vi "AddTopProcessRun.vi"(5 "ProcessRunStartTime (Now)":timestamp, 6 "ProcessRunStatus (NOT_COMPLETED)":T1=enum."NOT_COMPLETED", 7 "ProductFullName (Generic_Product)":string="Generic_Product", 8 "error in":errorcluster, 9 "ProductUnitIdentifier":string, 10 "ProcessFullName (Generic_Process)":string="Generic_Process", 11 "Datawarehouse in":refnum<class "Datawarehouse.lvclass">) -> (0 "error out":errorcluster, 2 "TopProcessRun":refnum<class "ProcessRun.lvclass">, 3 "Datawarehouse out":refnum<class "Datawarehouse.lvclass">)   [LabVIEW 2021, in "ProligentXMLGenerator.lvlib" / "Datawarehouse.lvclass"]
doc: "Add a Top Process Run.\n\nDefines a process run, a logical container for the execution of operations. Process runs are globaly unique by their ProcessRunId property."
uses:
  Datawarehouse.lvclass
  Datawarehouse.lvclass/Datawarehouse.ctl
  ProcessRun/ProcessRun.lvclass
  Base/ExecutionStatus/Value.ctl
  Base/ExecutionStatus/ExecutionStatus.lvclass
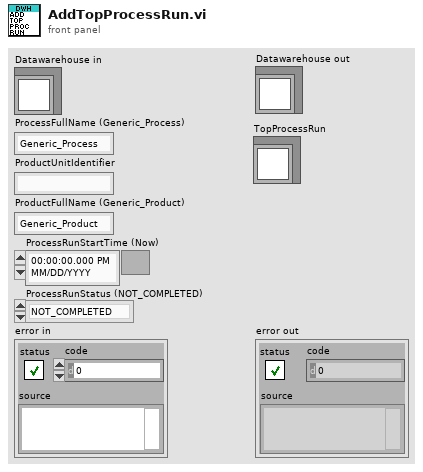
[diagram p1: front panel]
types:
  T1 = typedef "ProligentXMLGenerator.lvlib/ExecutionStatus.lvclass/Value.ctl" = enum16{"PASS", "FAIL", "NOT_COMPLETED", "ABORTED"}
  T2 = typedef "ProligentXMLGenerator.lvlib/Datawarehouse.lvclass/Data.ctl" = cluster{"DestinationFolder":path, "BaseFileName":string, "Document":refnum<k20>, "Defects":refnum<class "Defect.lvclass">[], "TopProcessRuns":refnum<class "ProcessRun.lvclass">[], "ProductUnits":refnum<class "ProductUnit.lvclass">[], "GenerationTime":refnum<class "DateTime.lvclass">, "DataSourceFingerprint":refnum<class "NonEmptyString_448.lvclass">, "IntegrationMetaData":refnum<class "NonEmptyString_2000.lvclass">, "TimeZoneInfoId":string}
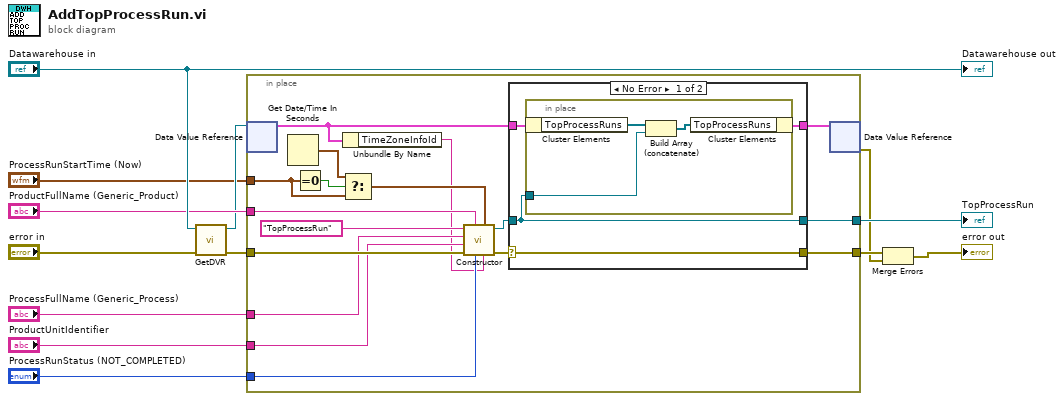
[diagram p0: block diagram]
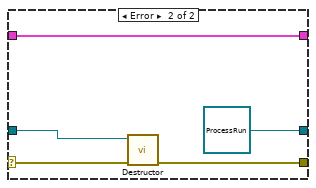
[diagram p2: hidden frame]
diagram:
  n1 = call "GetDVR.vi"("error in"="error in", "Datawarehouse"="Datawarehouse in") -> ("error out"=w4:errorcluster, "DVRReference"=w3:refnum<data-value>)  [unwired: 8 in]
  n2 = in-place "In Place Element Structure" {
    in-place-border: [w30] -> w5
    in-place-border: [w27] -> w13
    in-place-border: w4 -> [w26]
    in-place-border: "ProductFullName (Generic_Product)" -> [w24]
    in-place-border: "ProcessFullName (Generic_Process)" -> [w22]
    in-place-border: "ProductUnitIdentifier" -> [w21]
    in-place-border: "ProcessRunStatus (NOT_COMPLETED)" -> [w20]
    in-place-border: "ProcessRunStartTime (Now)" -> [w17]
    n3 = in-place-dvr #1(w3) -> (w15:T2)  [unwired: 1 out]
    n4 = Get Date/Time In Seconds() -> (seconds since 1Jan1904=w18:timestamp)
    n5 = Equal To 0?(x=w17) -> (x = 0?=w19:bool)
    n6 = Unbundle By Name(w15) -> ("TimeZoneInfoId"=w14:string)
    n7 = Select(t=w18, s=w19, f=w17) -> (s? t:f=w16:timestamp)
    n8 = call "Constructor.vi"("TimeZoneInfoId"=w14, "ProcessRunStartTime"=w16, "ProcessRunStatus"=w20, "ProductFullName"=w24, "error in"=w26, "ProductUnitIdentifier"=w21, "ProcessFullName"=w22, "Name"="TopProcessRun") -> ("error out"=w29:errorcluster, "ProcessRun out"=w28:refnum<class "ProcessRun.lvclass">)  [unwired: 2 in]
    n9 = case shown="No Error" w29 {
      selector: w29 -> [w34 w41]
      tunnel: w15 -> [w33 w42]
      tunnel: w28 -> [w31 w39]
      tunnel: [w32 w42] -> w25
      tunnel: [w34 w40] -> w30
      tunnel: [w31 refnum<class "ProcessRun.lvclass"> refnum ("TopProcessRun")] -> w27
      frame No Error {
        n10 = in-place "In Place Element Structure" {
          in-place-border: w31 -> [w35]
          n11 = in-place-cluster #2(w33) -> ("TopProcessRuns"=w37:refnum<class "ProcessRun.lvclass">[])
          n12 = Build Array (concatenate)(w37, w35) -> (w36:refnum<class "ProcessRun.lvclass">[])
          n13 = in-place-cluster #2("TopProcessRuns"=w36) -> (w32:T2)
        }
      }
      frame Error {
        n14 = call "Destructor.vi"("error in"=w41, "ProcessRun in"=w39) -> ("error out"=w40:errorcluster)  [unwired: 9 in]
      }
    }
    n15 = in-place-dvr #1(w25) -> (w2:errorcluster)  [unwired: 1 out]
  }
  "TopProcessRun" <- w13
  n16 = Merge Errors(w5, w2) -> (→"error out":errorcluster)
  "Datawarehouse out" <- "Datawarehouse in"
